vi "test_udp-w-joystick-old.vi"() -> ()   [LabVIEW 2019]
panel:
  in  "joystick scale":i32=327670
  in  "J-M":bool
  out "A_joystick":dbl=-0.0
  out "L_joystick":dbl=-0.0
  in  "local port":u16=61556
  in  "remote port":u16=61550
  in  "address":string="192.168.1.109"
  in  "Stop":bool=TRUE
  in  "dt":u32=50
  out "에러 출력":errorcluster
  out "s? t:f":string="H:L=-0.000000,A=-0.000000,"
  in  "A_a":dbl(slide) scale=-1.0..1.0
  in  "L_m":dbl(slide)=0.01412429378531073 scale=-0.1..0.1
  out "숫자형":i32=52702
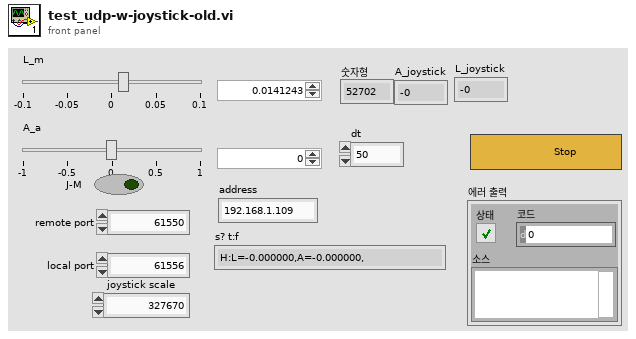
[diagram p1: front panel]
types:
  T1 = cluster{"axis info":cluster{"X axis":i32, "Y axis":i32, "Z axis":i32, "X axis rotation":i32, "Y axis rotation":i32, "Z axis rotation":i32, "U axis":i32, "V axis":i32}, "button info":cluster{"button 1":bool, "button 2":bool, "button 3":bool, "button 4":bool, "button 5":bool, "button 6":bool, "button 7":bool, "button 8":bool, "button 9":bool, "button 10":bool, "button 11":bool, "button 12":bool, "button 13":bool, "button 14":bool, "button 15":bool, "button 16":bool, "button 17":bool, "button 18":bool, "button 19":bool, "button 20":bool, "button 21":bool, "button 22":bool, "button 23":bool, "button 24":bool, "button 25":bool, "button 26":bool, "button 27":bool, "button 28":bool, "button 29":bool, "button 30":bool, "button 31":bool, "button 32":bool}, "direction info":cluster{"pov 1":i32, "pov 2":i32, "pov 3":i32, "pov 4":i32}}
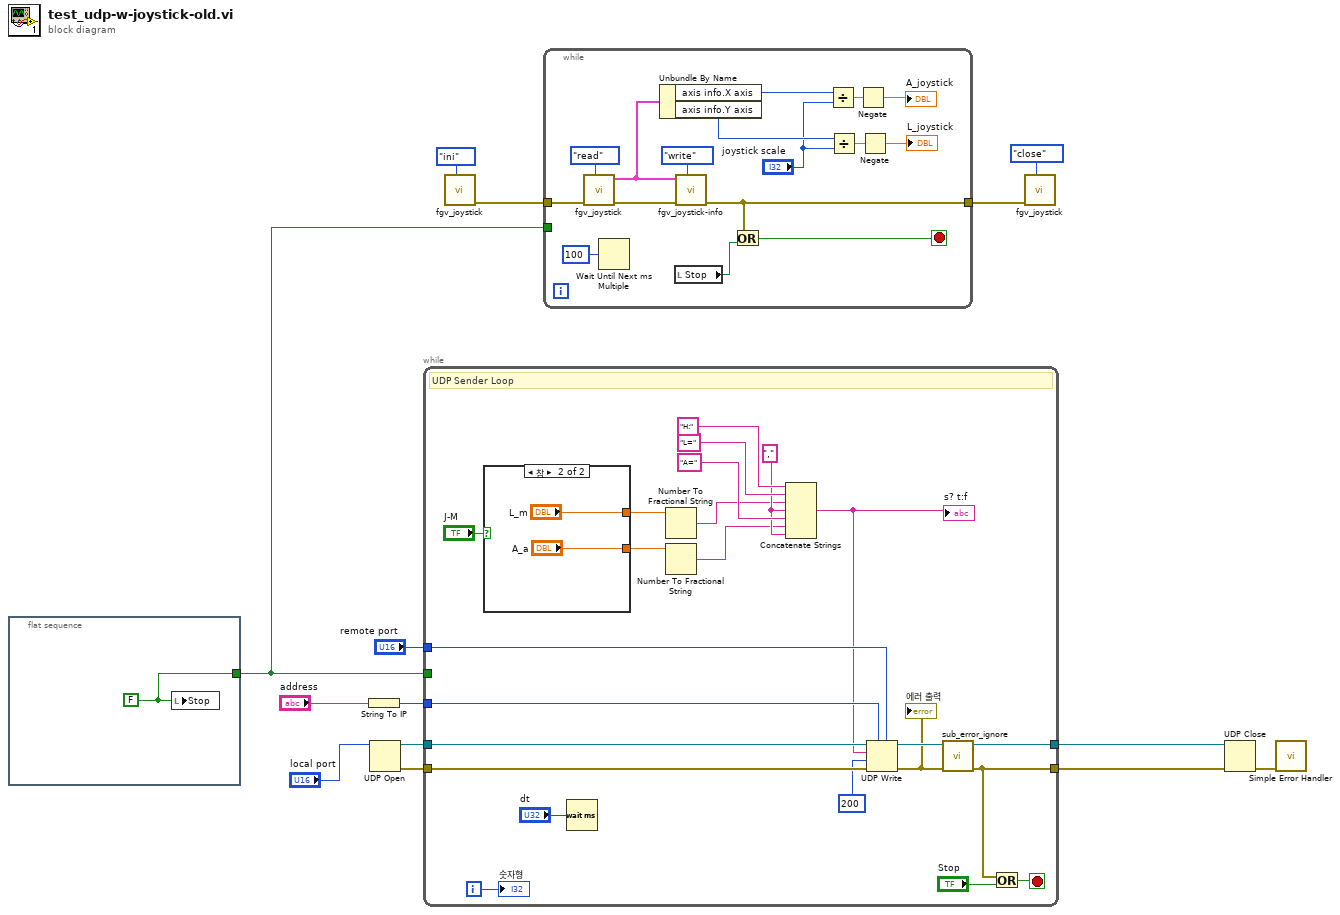
[diagram p0: block diagram]
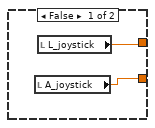
[diagram p2: hidden frame]
diagram:
  n1 = flat-sequence {
    tunnel: [w15] -> w1
    frame #0 {
      w15 = FALSE ("Stop")
      n2 = local write "Stop"(w15) -> ()
    }
  }
  n3 = String To IP(1:"address") -> (0:w10:u32)
  n4 = UDP Open(11:"local port") -> (port=w9:refnum<k16>, 0:w8:errorcluster)  [unwired: 4 in, 1 out]
  n5 = while {
    tunnel: [w27] -> w13
    tunnel: w9 -> [w37]
    tunnel: w8 -> [w36]
    tunnel: [w29] -> w14
    tunnel: w10 -> [w33]
    tunnel: "remote port" -> [w31]
    tunnel: w1 -> [_]
    i -> [w21]
    stop <- w35 stop-if-true
    w23 = ","
    # "UDP Sender Loop"
    n6 = case shown="참" "J-M" {
      tunnel: [w38 "A_a"] -> w19
      tunnel: [w39 "L_m"] -> w18
      frame False {
        n7 = local read "A_joystick"() -> (w38:dbl)
        n8 = local read "L_joystick"() -> (w39:dbl)
      }
      frame True {
      }
    }
    n9 = Wait (ms)(milliseconds to wait="dt") -> ()  [unwired: 1 out]
    n10 = Number To Fractional String(number=w18) -> (F-format string=w16:string)  [unwired: 3 in]
    n11 = Number To Fractional String(number=w19) -> (F-format string=w17:string)  [unwired: 3 in]
    n12 = Concatenate Strings("H:", "L=", w16, w23, "A=", w17, w23) -> (w22:string)
    "s? t:f" <- w22
    n13 = UDP Write(address=w33, port or service name=w31, connection ID=w37, data in=w22, 8:w36, 9:200 ("타임아웃 ms (25000)")) -> (error out=w28:errorcluster, 3:w29:refnum<k16>)
    "에러 출력" <- w28
    n14 = call "sub_error_ignore.vi"("error in"=w28) -> ("error out"=w27:errorcluster)  [unwired: 10 in]
    n15 = Or(x=w27, y="Stop") -> (x .or. y?=w35:bool)
    "숫자형" <- w21
  }
  n16 = call "fgv_joystick.vi"("cmd"=enum16{"ini", "read", "close"}."ini") -> ("error out"=w3:errorcluster)  [unwired: 9 in, 1 out]
  n17 = while {
    tunnel: w3 -> [w54]
    tunnel: [w52] -> w2
    tunnel: w1 -> [_]
    stop <- w55 stop-if-true
    n18 = call "fgv_joystick.vi"("cmd"=enum16{"ini", "read", "close"}."read", "error in"=w54) -> ("error out"=w53:errorcluster, "joystick info-out"=w49:T1)  [unwired: 8 in]
    n19 = Wait Until Next ms Multiple(millisecond multiple=u32 100 ("milliseconds to wait")) -> ()  [unwired: 1 out]
    n20 = Unbundle By Name(w49) -> ("axis info.X axis"=w48:i32, "axis info.Y axis"=w47:i32)
    n21 = local read "Stop"() -> (w50:bool)
    n22 = call "fgv_joystick-info.vi"("init"=enum16{"enable", "init", "read", "write"}."write", "error in"=w53, "joystick info-in"=w49) -> ("error out"=w52:errorcluster)  [unwired: 5 in, 3 out]
    n23 = Or(x=w52, y=w50) -> (x .or. y?=w55:bool)
    n24 = Divide(x=w48, y="joystick scale") -> (x/y=w45:dbl)
    n25 = Divide(x=w47, y="joystick scale") -> (x/y=w46:dbl)
    n26 = Negate(x=w45) -> (-x=→"A_joystick":dbl)
    n27 = Negate(x=w46) -> (-x=→"L_joystick":dbl)
  }
  n28 = call "fgv_joystick.vi"("cmd"=enum16{"ini", "read", "close"}."close", "error in"=w2) -> ()  [unwired: 8 in, 2 out]
  n29 = UDP Close(connection ID=w14, 8:w13) -> (error out=w11:errorcluster)  [unwired: 1 out]
  n30 = call <vilib>:"Simple Error Handler.vi"("error in (no error)"=w11) -> ()  [unwired: 4 in, 5 out]
